vi "Remove Name-Peroid.vi"(10 "Name":string, 11 "UserEventTimer in":refnum<class "TimerEngine.lvclass">) -> (2 "deleted timePeroid":i32, 3 "UserEventTimer out":refnum<class "TimerEngine.lvclass">)   [LabVIEW 2017, in "TimerEngine.lvlib" / "TimerEngine.lvclass"]
uses:
  TimerEngine.lvclass
  TimerEngine.lvclass/TimerEngine.ctl
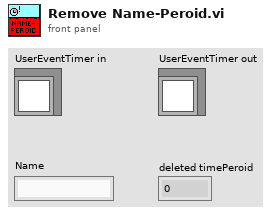
[diagram p1: front panel]
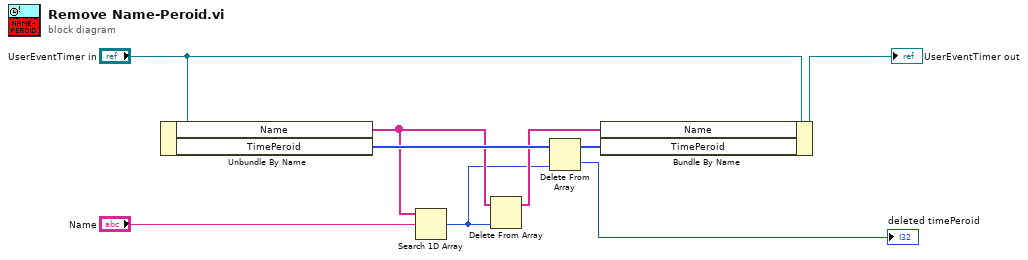
[diagram p0: block diagram]
diagram:
  n1 = Unbundle By Name("UserEventTimer in") -> ("Name"=w4:string[], "TimePeroid"=w7:i32[])
  n2 = Search 1D Array(1D array=w4, element="Name") -> (index of element=w2:i32)  [unwired: 1 in]
  n3 = Delete From Array(array=w4, index=w2) -> (array with subset deleted=w3:string[])  [unwired: 1 in, 1 out]
  n4 = Delete From Array(array=w7, index=w2) -> (deleted portion=→"deleted timePeroid":i32, array with subset deleted=w5:i32[])  [unwired: 1 in]
  n5 = Bundle By Name(cluster="UserEventTimer in", "Name"=w3, "TimePeroid"=w5) -> (→"UserEventTimer out":refnum<class "TimerEngine.lvclass">)
